vi "SegmentNameAdjustment.vi"(8 "Right":string, 9 "Left":string, 10 "Segment In":string, 11 "Activity":bool) -> (2 "Segment Out":string)   [LabVIEW 2013, in "main.lvlib"]
uses:
  main.lvlib
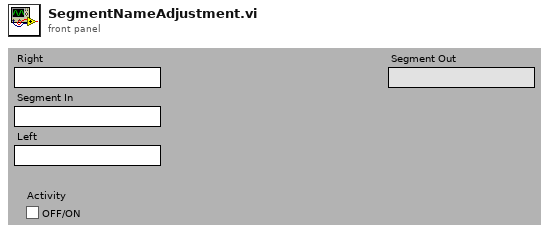
[diagram p1: front panel]
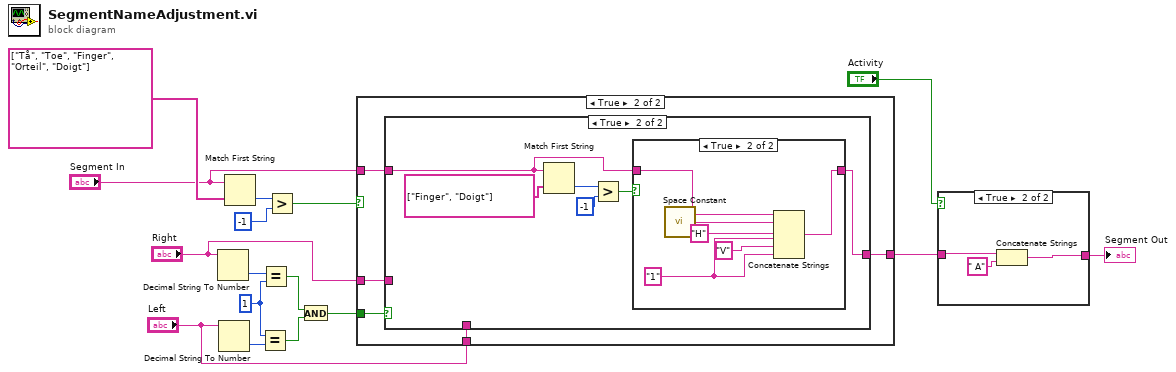
[diagram p0: block diagram]
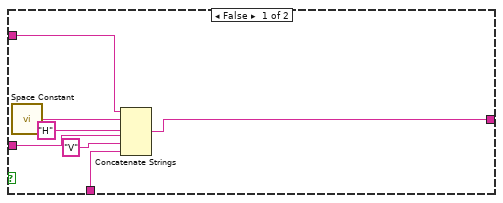
[diagram p4: hidden frame]
diagram:
  w8 = 1
  n1 = Decimal String To Number(string="Right") -> (number=w10:i32)  [unwired: 2 in, 1 out]
  n2 = Decimal String To Number(string="Left") -> (number=w9:i32)  [unwired: 2 in, 1 out]
  n3 = Match First String(2:string[] ["Tå", "Toe", "Finger", "Orteil", "Doigt"], 3:"Segment In") -> (0:w5:i32)  [unwired: 1 out]
  n4 = Equal?(x=w8, y=w9) -> (x = y?=w6:bool)
  n5 = Equal?(x=w10, y=w8) -> (x = y?=w7:bool)
  n6 = Greater?(x=w5, y=-1) -> (0:w11:bool)
  n7 = And(x=w7, y=w6) -> (x .and. y?=w16:bool)
  n8 = case shown="True" w11 {
    tunnel: [w17 w22] -> w2
    tunnel: w16 -> [_ w21]
    tunnel: "Right" -> [_ w20]
    tunnel: "Left" -> [_ w19]
    tunnel: "Segment In" -> [w17 w18]
    frame False {
    }
    frame True {
      n9 = case shown="True" w21 {
        tunnel: [w28 w31] -> w22
        tunnel: w18 -> [w27 w30]
        tunnel: w20 -> [w25 _]
        tunnel: w19 -> [w23 _]
        frame False {
          n10 = call <vilib>:"Space Constant.vi"() -> ("String"=w29:string)
          n11 = Concatenate Strings(w27, w29, "H", w25, "V", w23) -> (w28:string)
        }
        frame True {
          n12 = Match First String(2:string[] ["Finger", "Doigt"] ("string array"), 3:w30) -> (0:w34:i32)  [unwired: 1 out]
          n13 = Greater?(x=w34, y=-1) -> (0:w32:bool)
          n14 = case shown="True" w32 {
            tunnel: w30 -> [w36 w39]
            tunnel: [w36 w38] -> w31
            frame False {
            }
            frame True {
              w37 = "1"
              n15 = call <vilib>:"Space Constant.vi"() -> ("String"=w42:string)
              n16 = Concatenate Strings(w39, w42, "H", w37, "V", w37) -> (w38:string)
            }
          }
        }
      }
    }
  }
  n17 = case shown="True" "Activity" {
    tunnel: w2 -> [w43 w46]
    tunnel: [w43 w44] -> w1
    frame False {
    }
    frame True {
      n18 = Concatenate Strings(w46, " A" ("string")) -> (w44:string)
    }
  }
  "Segment Out" <- w1
